vi "Periodic Tasks.vi"(8 "error in":errorcluster) -> ()   [LabVIEW 2014]
doc: "This VI runs in parallel to other tasks. It can contain as many user-defined periodic loops as you need. These can carry out PID or other sorts of timed response."
uses:
  <vilib>/Rock Robotics/WPI/DriverStation/WPI_DriverStationRobotMode2.ctl
  Robot Global Data.vi
  Utilities/CanGrabberSetpoint.vi
  <vilib>/Rock Robotics/Network Tables/SD Read Number.vi
  Automated Tasks/AutomationGlobals.vi
  <vilib>/Rock Robotics/Network Tables/SD Write Boolean.vi
  Automated Tasks/ToteCount.vi
  <vilib>/Rock Robotics/Network Tables/SD Write Number.vi
  <vilib>/Rock Robotics/WPI/Compressor/WPI_CompressorGetSetRefNum.vi
panel:
  out "Right Can Grabber POS":dbl
  out "Left Can Grabber POS":dbl
  out "AutoMode":dbl
  # "Kc = 100, Kd = 37 - 1/15/2015"
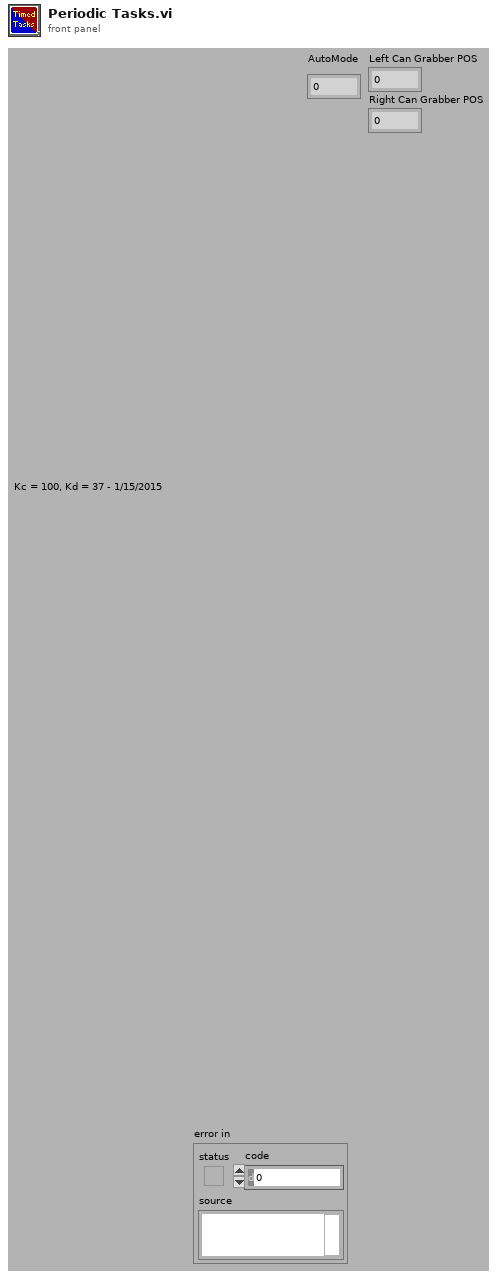
[diagram p1: front panel]
types:
  T1 = typedef "WPI_DriverStationRobotMode2.ctl" = enum16{"Autonomous Disabled", "Autonomous Enabled", "Teleop Disabled", "Teleop Enabled", "Disconnected", "Finish", "Test Disabled", "Test Enabled", "Emergency Stopped"}
  T2 = typedef "WPI_MotorControlDeviceRef.ctl" = cluster{"DeviceStatus":errorcluster, "Type":T3, "PWM":cluster{"Controller":T4, "PWM Channel":T5, "DeadBand":T6}, "CAN":cluster{"Device Number":u8, "Control Mode":T7, "Semaphore":T8, "Max Vout":dbl, "TalonSRX Control Mode":T9}, "Invert":bool, "TransformRef":T10, "InvTransformRef":T10}
  T3 = typedef "WPI_MotorControlType.ctl" = enum16{"PWM", "CAN", "CANTalonSRX"}
  T4 = typedef "FPGA_TypedefDigitalModule.ctl" = enum16{"Controller 1"}
  T5 = typedef "FPGA_DIOPWMChannel.ctl" = enum8{"PWM 0", "PWM 1", "PWM 2", "PWM 3", "PWM 4", "PWM 5", "PWM 6", "PWM 7", "PWM 8", "PWM 9", "PWM MXP 0", "PWM MXP 1", "PWM MXP 2", "PWM MXP 3", "PWM MXP 4", "PWM MXP 5", "PWM MXP 6", "PWM MXP 7", "PWM MXP 8", "PWM MXP 9", "Invalid"}
  T6 = typedef "WPI_PWMDeadband.ctl" = cluster{"Name":string, "maxPositivePwm":i32, "minPositivePwm":i32, "centerPwm":i32, "maxNegativePwm":i32, "minNegativePwm":i32, "angularRange":u16}
  T7 = typedef "WPI_CANJaguar_ControlMode.ctl" = enum8{"Percent VBus", "Current", "Speed", "Position", "Voltage"}
  T8 = typedef "Semaphore RefNum" = refnum<k1>
  T9 = typedef "WPI_CANTalonSRX_APIControlMode.ctl" = enum8{"Percent VBus", "Speed", "Position", "Slave", "Unchanged / Invalid"}
  T10 = typedef "WPI_PWMTransform_ConPane.ctl" = refnum<vi>
  T11 = typedef "WPI_CANTalonSRX_GlobalStatus.ctl" = cluster{"Applied Throttle":dbl, "Module Enabled":bool, "CAN Error":errorcluster, "Closed Loop Error":dbl, "Forward Limit Switch Closed":bool, "Reverse Limit Switch Closed":bool, "Sensor Position":dbl, "Sensor Velocity":dbl, "Current":dbl, "Sticky Fault - Over Temp":bool, "Sticky Fault - Under Voltage":bool, "Sticky Fault - Forward Limit":bool, "Sticky Fault - Reverse Limit":bool, "Sticky Fault - Forward Soft Limit":bool, "Sticky Fault - Reverse Soft Limit":bool, "Brake is Enabled":bool, "Encoder Position":dbl, "Encoder Velocity":dbl, "Encoder Index Count":dbl, "Encoder A Pin State":bool, "Encoder B Pin State":bool, "Encoder Index Pin State":bool, "Analog In":dbl, "Analog In Velocity":dbl, "Temperature (C)":dbl, "Battery Voltage":dbl}
  T12 = typedef "WPI_CompressorDevRef.ctl" = cluster{"DevStatus":errorcluster, "Pneumatics Control Module":u8}
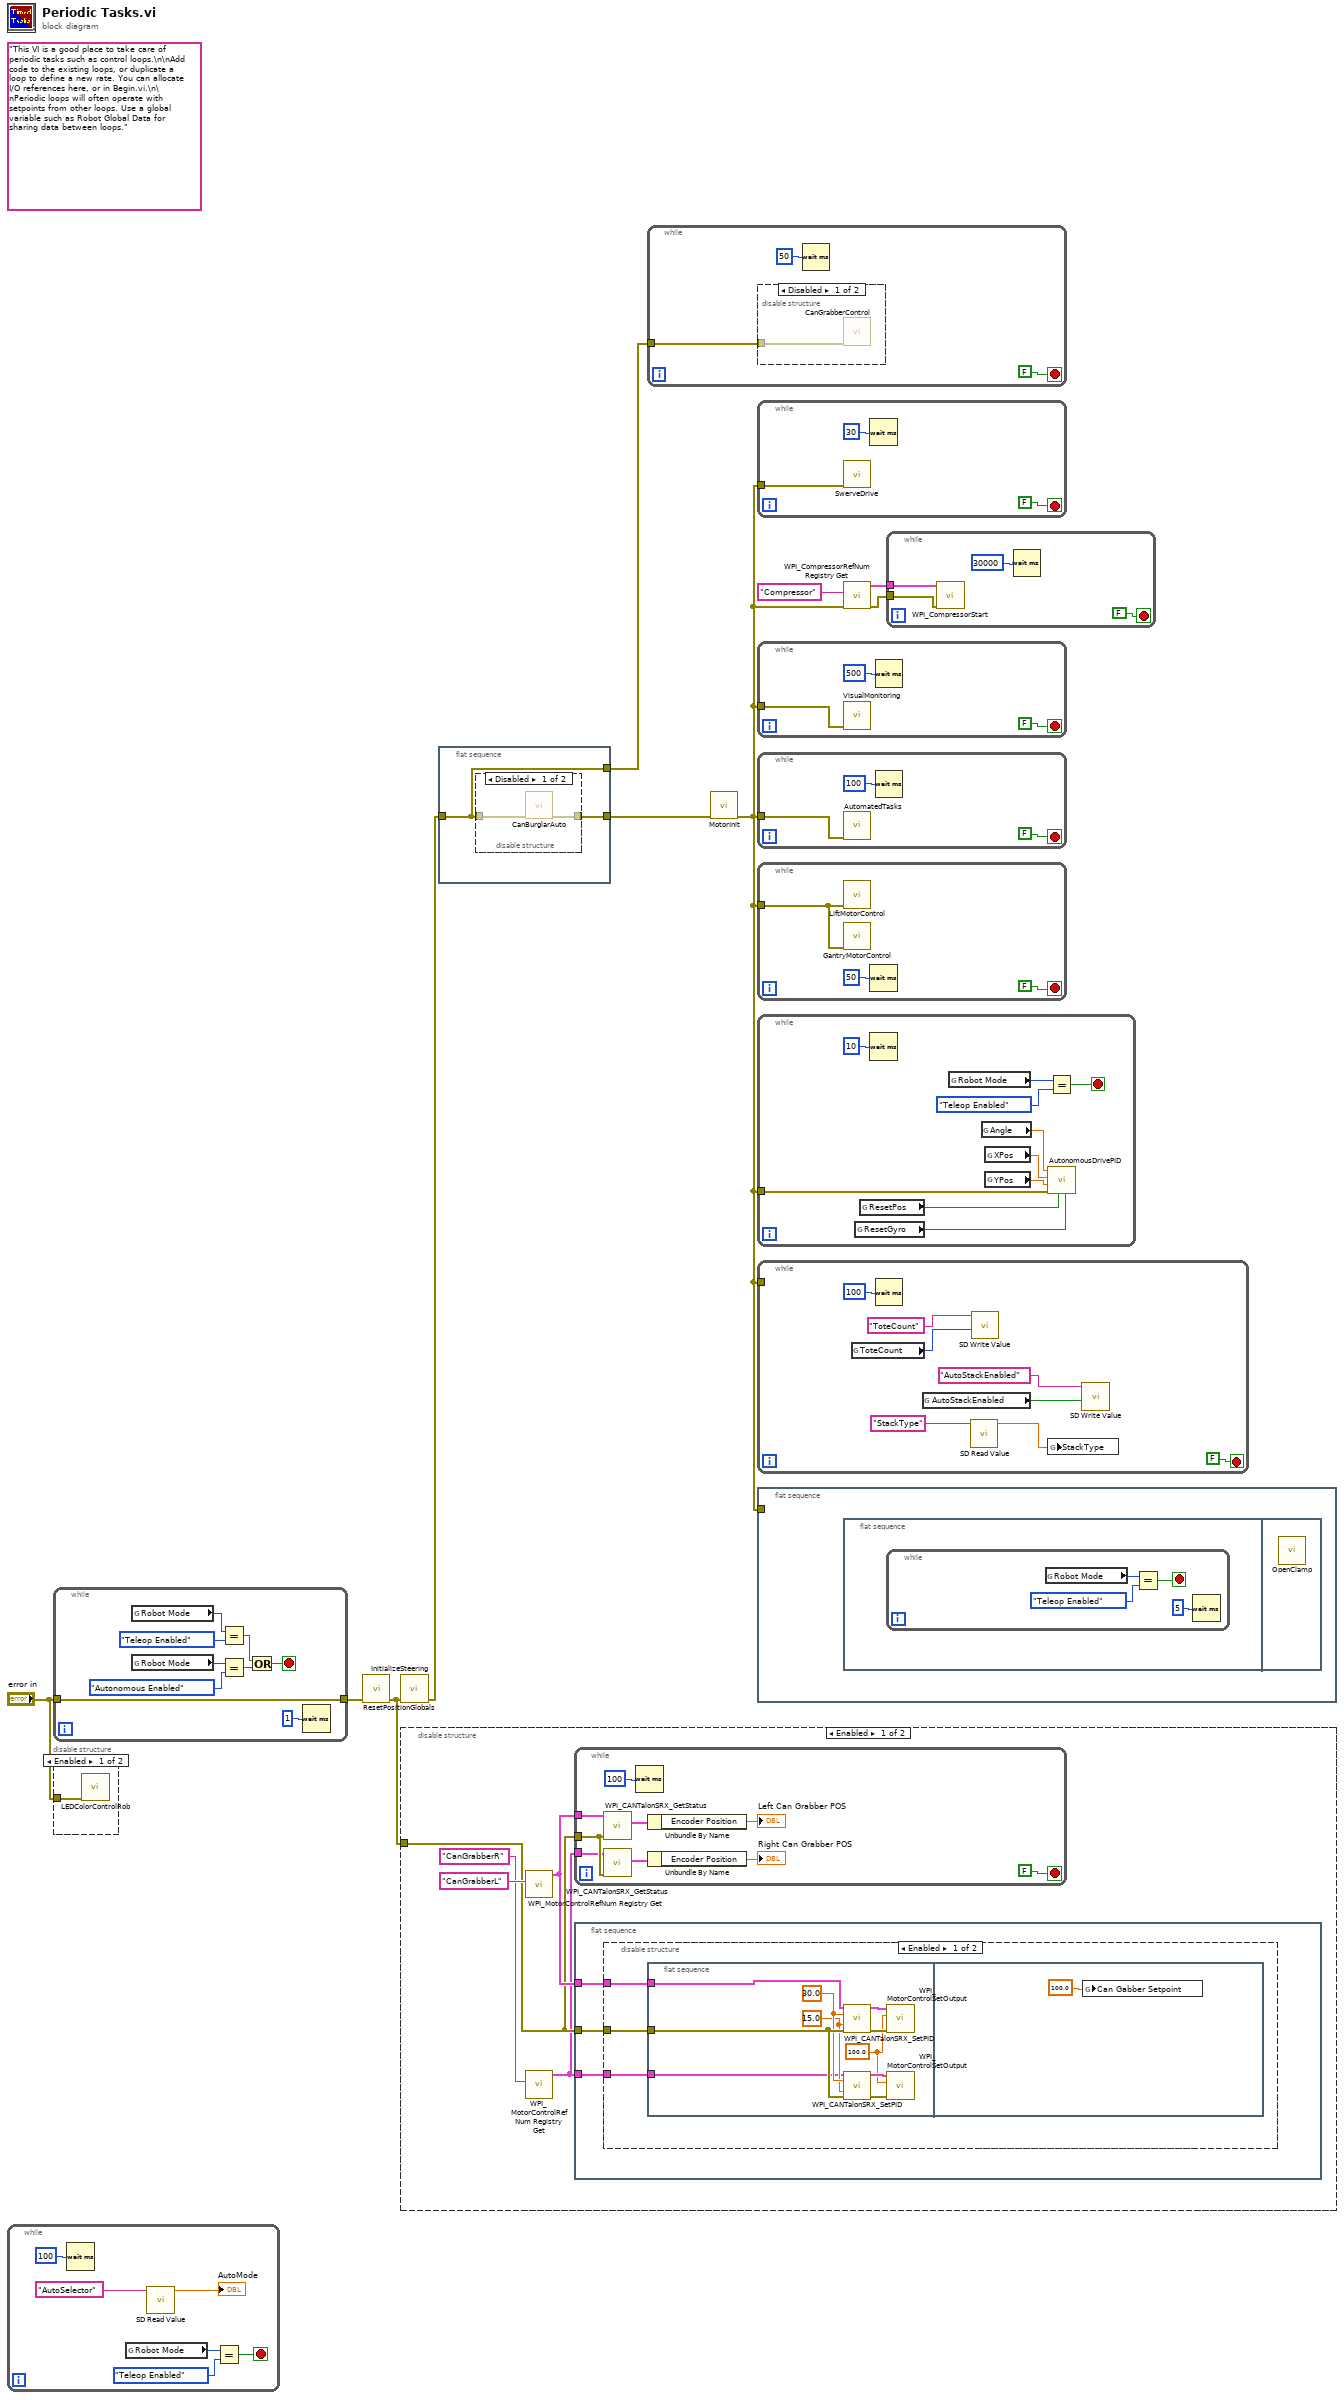
[diagram p0: block diagram]
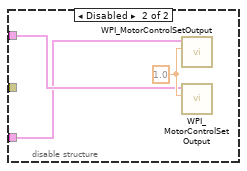
[diagram p3: hidden frame]
diagram:
  (unwired) "This VI is a good place to take care of periodic tasks such as control loops.\n\nAdd code to the existing loops, or duplicate a loop to define a new rate. You can allocate I/O references here, or in Begin.vi.\n\nPeriodic loops will often operate with setpoints from other loops. Use a global variable such as Robot Global Data for sharing data between loops."
  n1 = while {
    stop <- w11 stop-if-true
    n2 = Wait (ms)(milliseconds to wait=u32 100) -> ()  [unwired: 1 out]
    n3 = global read "Robot Global Data.vi" "Robot Mode"() -> (w13:T1)
    n4 = call-poly <vilib>:"SD Read Value.vi"("Name"="AutoSelector") -> ("Numeric"=→"AutoMode":dbl)  [unwired: 8 in, 2 out]
    n5 = Equal?(x=w13, y=WPI_DriverStationRobotMode2."Teleop Enabled") -> (x = y?=w11:bool)
  }
  n6 = while {
    tunnel: "error in" -> [w18]
    tunnel: [w18] -> w6
    stop <- w19 stop-if-true
    n7 = global read "Robot Global Data.vi" "Robot Mode"() -> (w25:T1)
    n8 = global read "Robot Global Data.vi" "Robot Mode"() -> (w23:T1)
    n9 = Equal?(x=w25, y=WPI_DriverStationRobotMode2."Teleop Enabled") -> (x = y?=w21:bool)
    n10 = Equal?(x=w23, y=WPI_DriverStationRobotMode2."Autonomous Enabled") -> (x = y?=w20:bool)
    n11 = Or(x=w21, y=w20) -> (x .or. y?=w19:bool)
    n12 = Wait (ms)(milliseconds to wait=u32 1) -> ()  [unwired: 1 out]
  }
  n13 = disable-structure shown="Enabled" {
    disable-tunnel: "error in" -> [w26 _]
    frame Enabled {
      n14 = call "LEDColorControlRob.vi"("error in"=w26) -> ()  [unwired: 11 in]
    }
    frame Disabled {
    }
  }
  n15 = call "ResetPositionGlobals.vi"("error in"=w6) -> ("error out"=w4:errorcluster)  [unwired: 10 in]
  n16 = call "InitializeSteering.vi"("error in (no error)"=w4) -> ("error out"=w5:errorcluster)  [unwired: 10 in]
  n17 = disable-structure shown="Enabled" {
    disable-tunnel: w4 -> [w29 _]
    frame Enabled {
      n18 = call <vilib>:"WPI_MotorControlRefNum Registry Get.vi"("refnum name"="CanGrabberL") -> ("MotorControlDevRef"=w30:T2)  [unwired: 9 in, 1 out]
      n19 = call <vilib>:"WPI_MotorControlRefNum Registry Get.vi"("refnum name"="CanGrabberR") -> ("MotorControlDevRef"=w27:T2)  [unwired: 9 in, 1 out]
      n20 = while {
        tunnel: w30 -> [w40]
        tunnel: w29 -> [w35]
        tunnel: w27 -> [w34]
        stop <- FALSE stop-if-true
        n21 = call <vilib>:"WPI_CANTalonSRX_GetStatus.vi"("error in (no error)"=w35, "CAN Talon SRX Ref"=w40) -> ("Talon SRX Status"=w39:T11)  [unwired: 7 in, 2 out]
        n22 = call <vilib>:"WPI_CANTalonSRX_GetStatus.vi"("error in (no error)"=w35, "CAN Talon SRX Ref"=w34) -> ("Talon SRX Status"=w33:T11)  [unwired: 7 in, 2 out]
        n23 = Wait (ms)(milliseconds to wait=u32 100) -> ()  [unwired: 1 out]
        n24 = Unbundle By Name(w39) -> ("Encoder Position"=→"Left Can Grabber POS":dbl)
        n25 = Unbundle By Name(w33) -> ("Encoder Position"=→"Right Can Grabber POS":dbl)
      }
      n26 = flat-sequence {
        tunnel: w29 -> [w42]
        tunnel: w30 -> [w43]
        tunnel: w27 -> [w41]
        frame #0 {
          n27 = disable-structure shown="Enabled" {
            disable-tunnel: w43 -> [w46 w59]
            disable-tunnel: w42 -> [w45 _]
            disable-tunnel: w41 -> [w44 w58]
            frame Enabled {
              n28 = flat-sequence {
                tunnel: w46 -> [w56]
                tunnel: w45 -> [w55]
                tunnel: w44 -> [w52]
                frame #0 {
                  w47 = 100.0 ("Output")
                  w53 = 15.0 ("D")
                  w54 = 30.0 ("P")
                  n29 = call <vilib>:"WPI_CANTalonSRX_SetPID.vi"("CAN Talon SRX Ref"=w56, "P"=w54, "D"=w53, "error in (no error)"=w55) -> ("CAN Talon SRX Ref Out"=w50:T2, "error out"=w51:errorcluster)  [unwired: 10 in]
                  n30 = call <vilib>:"WPI_CANTalonSRX_SetPID.vi"("CAN Talon SRX Ref"=w52, "P"=w54, "D"=w53, "error in (no error)"=w55) -> ("CAN Talon SRX Ref Out"=w49:T2, "error out"=w48:errorcluster)  [unwired: 10 in]
                  n31 = call <vilib>:"WPI_MotorControlSetOutput.vi"("error in (no error)"=w51, "Output"=w47, "MotorControlDevRef"=w50) -> ()  [unwired: 6 in, 3 out]
                  n32 = call <vilib>:"WPI_MotorControlSetOutput.vi"("error in (no error)"=w48, "Output"=w47, "MotorControlDevRef"=w49) -> ()  [unwired: 6 in, 3 out]
                }
                frame #1 {
                  n33 = global write "CanGrabberSetpoint.vi" "Can Gabber Setpoint"(100.0 ("Output")) -> ()
                }
              }
            }
            frame Disabled {
              w60 = 1.0 ("Output")
              n34 = call <vilib>:"WPI_MotorControlSetOutput.vi"("Output"=w60, "MotorControlDevRef"=w58) -> ()  [unwired: 7 in, 3 out]
              n35 = call <vilib>:"WPI_MotorControlSetOutput.vi"("Output"=w60, "MotorControlDevRef"=w59) -> ()  [unwired: 7 in, 3 out]
            }
          }
        }
      }
    }
    frame Disabled {
    }
  }
  n36 = flat-sequence {
    tunnel: w5 -> [w61]
    tunnel: [w62] -> w3
    tunnel: [w61] -> w2
    frame #0 {
      n37 = disable-structure shown="Disabled" {
        disable-tunnel: [w64 _] -> w62
        disable-tunnel: w61 -> [w63 _]
        frame Disabled {
          n38 = call "CanBurglarAuto.vi"("error in"=w63) -> ("error out"=w64:errorcluster)  [unwired: 10 in]
        }
        frame Enabled {
        }
      }
    }
  }
  n39 = while {
    tunnel: w2 -> [w65]
    stop <- FALSE stop-if-true
    n40 = disable-structure shown="Disabled" {
      disable-tunnel: w65 -> [w68 _]
      frame Disabled {
        n41 = call "CanGrabberControl.vi"("error in"=w68) -> ()  [unwired: 11 in]
      }
      frame Enabled {
      }
    }
    n42 = Wait (ms)(milliseconds to wait=u32 50) -> ()  [unwired: 1 out]
  }
  n43 = call "MotorInit.vi"("error in"=w3) -> ("error out"=w1:errorcluster)  [unwired: 10 in]
  n44 = while {
    tunnel: w1 -> [w69]
    stop <- FALSE stop-if-true
    n45 = call "SwerveDrive.vi"("error in (no error)"=w69) -> ()  [unwired: 11 in]
    n46 = Wait (ms)(milliseconds to wait=u32 30) -> ()  [unwired: 1 out]
  }
  n47 = while {
    tunnel: w1 -> [w72]
    stop <- FALSE stop-if-true
    n48 = call "VisualMonitoring.vi"("error in"=w72) -> ()  [unwired: 11 in]
    n49 = Wait (ms)(milliseconds to wait=u32 500) -> ()  [unwired: 1 out]
  }
  n50 = while {
    tunnel: w1 -> [w75]
    stop <- FALSE stop-if-true
    n51 = call "AutomatedTasks.vi"("error in"=w75) -> ()  [unwired: 11 in]
    n52 = Wait (ms)(milliseconds to wait=u32 100) -> ()  [unwired: 1 out]
  }
  n53 = while {
    tunnel: w1 -> [w78]
    stop <- FALSE stop-if-true
    n54 = call "LiftMotorControl.vi"("error in"=w78) -> ()  [unwired: 11 in]
    n55 = call "GantryMotorControl.vi"("error in"=w78) -> ()  [unwired: 11 in]
    n56 = Wait (ms)(milliseconds to wait=u32 50) -> ()  [unwired: 1 out]
  }
  n57 = while {
    tunnel: w1 -> [w90]
    stop <- w81 stop-if-true
    n58 = global read "AutomationGlobals.vi" "ResetGyro"() -> (w87:bool)
    n59 = global read "AutomationGlobals.vi" "ResetPos"() -> (w88:bool)
    n60 = Wait (ms)(milliseconds to wait=u32 10) -> ()  [unwired: 1 out]
    n61 = global read "Robot Global Data.vi" "Robot Mode"() -> (w83:T1)
    n62 = global read "AutomationGlobals.vi" "Angle"() -> (w85:dbl)
    n63 = global read "AutomationGlobals.vi" "XPos"() -> (w86:dbl)
    n64 = global read "AutomationGlobals.vi" "YPos"() -> (w84:dbl)
    n65 = Equal?(x=w83, y=WPI_DriverStationRobotMode2."Teleop Enabled") -> (x = y?=w81:bool)
    n66 = call "AutonomousDrivePID.vi"("ResetGyro"=w87, "ResetPosition"=w88, "error in (no error)"=w90, "YSetpoint"=w84, "XSetpoint"=w86, "AngleSetpoint"=w85) -> ()  [unwired: 6 in]
  }
  n67 = while {
    tunnel: w1 -> [_]
    stop <- FALSE stop-if-true
    n68 = global read "ToteCount.vi" "ToteCount"() -> (w93:i32)
    n69 = Wait (ms)(milliseconds to wait=u32 100) -> ()  [unwired: 1 out]
    n70 = global read "AutomationGlobals.vi" "AutoStackEnabled"() -> (w96:bool)
    n71 = call-poly <vilib>:"SD Read Value.vi"("Name"="StackType") -> ("Numeric"=w91:dbl)  [unwired: 8 in, 2 out]
    n72 = call-poly <vilib>:"SD Write Value.vi"("Numeric"=w93, "Name"="ToteCount") -> ()  [unwired: 8 in, 2 out]
    n73 = global write "AutomationGlobals.vi" "StackType"(w91) -> ()
    n74 = call-poly <vilib>:"SD Write Value.vi"("Boolean"=w96, "Name"="AutoStackEnabled") -> ()  [unwired: 8 in, 2 out]
  }
  n75 = flat-sequence {
    tunnel: w1 -> [_]
    frame #0 {
      n76 = flat-sequence {
        frame #0 {
          n77 = while {
            stop <- w100 stop-if-true
            n78 = global read "Robot Global Data.vi" "Robot Mode"() -> (w102:T1)
            n79 = Equal?(x=w102, y=WPI_DriverStationRobotMode2."Teleop Enabled") -> (x = y?=w100:bool)
            n80 = Wait (ms)(milliseconds to wait=u32 5) -> ()  [unwired: 1 out]
          }
        }
        frame #1 {
          n81 = call "OpenClamp.vi"() -> ()  [unwired: 12 in]
        }
      }
    }
  }
  n82 = call <vilib>:"WPI_CompressorRefNum Registry Get.vi"("error in (no error)"=w1, "refnum name"="Compressor") -> ("error out"=w8:errorcluster, "CompressorDevRef"=w9:T12)  [unwired: 8 in]
  n83 = while {
    tunnel: w9 -> [w104]
    tunnel: w8 -> [w103]
    stop <- FALSE stop-if-true
    n84 = call <vilib>:"WPI_CompressorStart.vi"("error in (no error)"=w103, "CompressorDevRef"=w104) -> ()  [unwired: 8 in, 2 out]
    n85 = Wait (ms)(milliseconds to wait=u32 30000) -> ()  [unwired: 1 out]
  }
